vi "whichLasersForAcq_v1.vi"(2 "LSFM_3 lasers":T1(array[cluster])=[{"Component ID"="405nm", "COM Port"="COM14", "Type "=enum."omicronLuxX", "init"=0, "Max power (mW)"=60.0}, {"Component ID"="488nm", "COM Port"="COM4", "Type "=enum."omicronLuxX", "init"=0, "Max power (mW)"=60.0}, {"Component ID"="561nm", "COM Port"="COM27", "Type "=enum."coherentObis", "init"=0, "Max power (mW)"=50.0}, {"Component ID"="642nm", "COM Port"="COM12", "Type "=enum."omicronLuxX", "init"=0, "Max power (mW)"=140.0}], 6 "405 nm (aq)":bool=TRUE, 7 "405 filter":u8(ring)=1 items=["460/36 [DAPI]"=1, "525/50 [FITC]"=2, "605/70 [Cy3]"=3, "665/LP [Cy5]"=4, "Empty-1"=5, "Empty-2"=6], 8 "488 nm (aq)":bool=TRUE, 9 "488 filter":u8(ring)=2 items=["460/36 [DAPI]"=1, "525/50 [FITC]"=2, "605/70 [Cy3]"=3, "665/LP [Cy5]"=4, "Empty-1"=5, "Empty-2"=6], 10 "561 nm (aq)":bool=TRUE, 11 "561 filter":u8(ring)=3 items=["460/36 [DAPI]"=1, "525/50 [FITC]"=2, "605/70 [Cy3]"=3, "665/LP [Cy5]"=4, "Empty-1"=5, "Empty-2"=6], 12 "642 nm (aq)":bool=TRUE, 13 "642 filter":u8(ring)=4 items=["460/36 [DAPI]"=1, "525/50 [FITC]"=2, "605/70 [Cy3]"=3, "665/LP [Cy5]"=4, "Empty-1"=5, "Empty-2"=6]) -> (16 "initLasers":T1(array[cluster]), 17 "initFilters":u8[](array[ring]) items=["460/36 [DAPI]"=1, "525/50 [FITC]"=2, "605/70 [Cy3]"=3, "665/LP [Cy5]"=4, "Empty-1"=5, "Empty-2"=6])   [LabVIEW 2015]
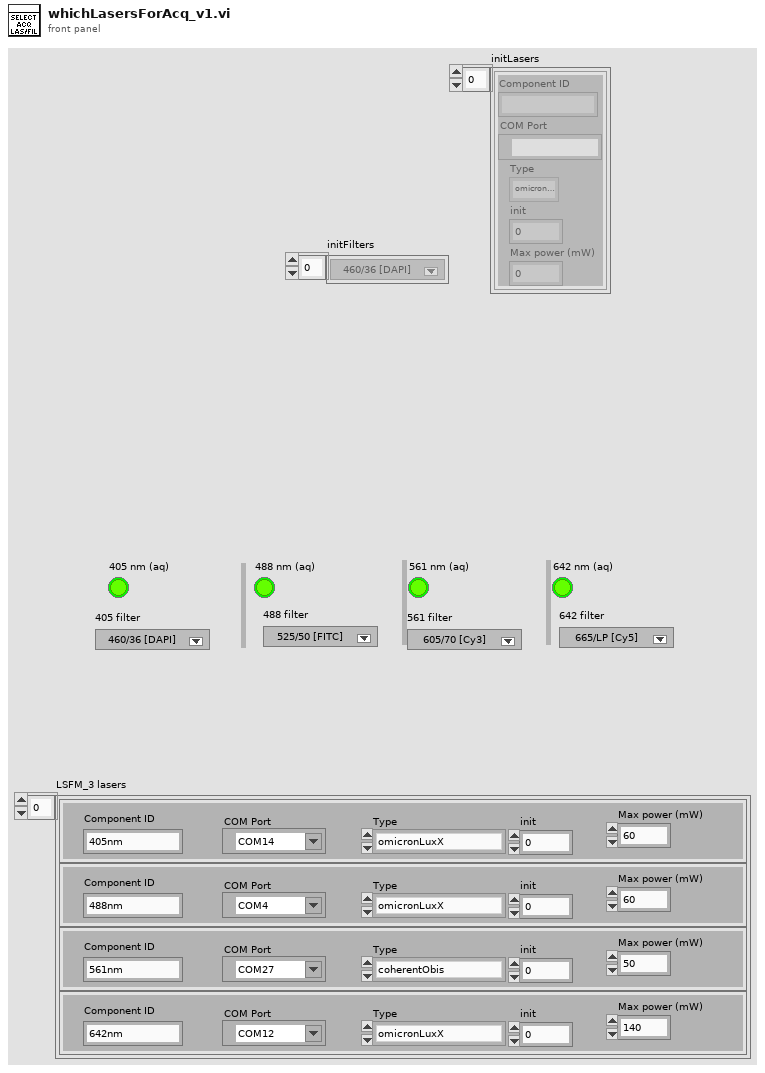
[diagram p1: front panel]
types:
  T1 = cluster{"Component ID":string, "COM Port":refnum<visa-resource-name>, "Type ":enum16{"omicronLuxX", "coherentObis"}, "init":i16, "Max power (mW)":dbl}[]
  T2 = cluster{"Component ID":string, "COM Port":refnum<visa-resource-name>, "Type ":enum16{"omicronLuxX", "coherentObis"}, "init":i16, "Max power (mW)":dbl}
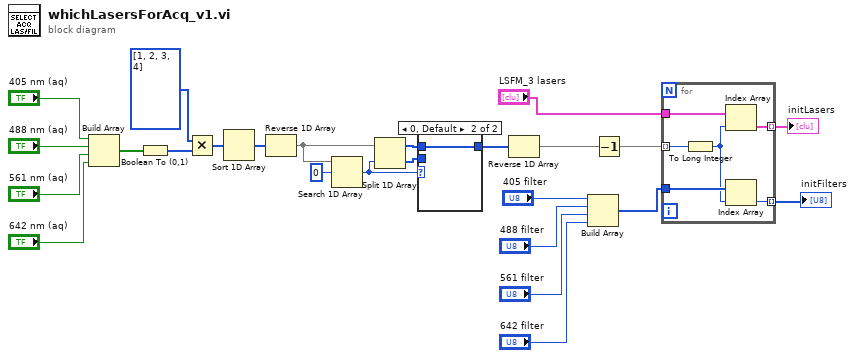
[diagram p0: block diagram]
diagram:
  n1 = Build Array("405 nm (aq)", "488 nm (aq)", "561 nm (aq)", "642 nm (aq)") -> (w9:bool[])
  n2 = Boolean To (0,1)(Boolean=w9) -> (0, 1=w24:i16[])
  n3 = Multiply(x=i16[] [1, 2, 3, 4], y=w24) -> (x*y=w25:i16[])
  n4 = Sort 1D Array(array=w25) -> (sorted array=w19:i16[])
  n5 = Reverse 1D Array(array=w19) -> (reversed array=w20:i16[])
  n6 = Search 1D Array(1D array=w20, element=i16 0) -> (index of element=w21:i32)  [unwired: 1 in]
  n7 = Split 1D Array(array=w20, index=w21) -> (first subarray=w22:i16[], second subarray=w23:i16[])
  n8 = case shown="0, Default" w21 {
    tunnel: w22 -> [_ w27]
    tunnel: w23 -> [w26 _]
    tunnel: [w26 w27] -> w17
    frame -1 {
    }
    frame 0, Default {
    }
  }
  n9 = Reverse 1D Array(array=w17) -> (reversed array=w18:i16[])
  n10 = Build Array("405 filter", "488 filter", "561 filter", "642 filter") -> (w15:u8[])
  n11 = Decrement(x=w18) -> (x-1=w16:i16[])
  n12 = for {
    tunnel: w16 -> [w29] mode=indexing
    tunnel: "LSFM_3 lasers" -> [w33]
    tunnel: [w32] -> w1 mode=indexing
    tunnel: w15 -> [w31]
    tunnel: [w30] -> w3 mode=indexing
    n13 = To Long Integer(number=w29) -> (32bit integer=w28:i32)
    n14 = Index Array(array=w33, index=w28) -> (element=w32:T2)
    n15 = Index Array(array=w31, index=w28) -> (element=w30:u8)
  }
  "initFilters" <- w3
  "initLasers" <- w1
